vi "GetType.vi"(8 "error in (no error)":errorcluster, 11 "Configure Alarms Msg":refnum<class "Configure Alarms Msg.lvclass">) -> (0 "error out":errorcluster, 2 "Data Sample":variant, 3 "Configure Alarms Msg":refnum<class "Configure Alarms Msg.lvclass">)   [LabVIEW 2015, in "LS218.lvlib" / "Configure Alarms Msg.lvclass"]
uses:
  Configure Alarms Msg.lvclass
  Configure Alarms Msg.lvclass/Configure Alarms Msg.ctl
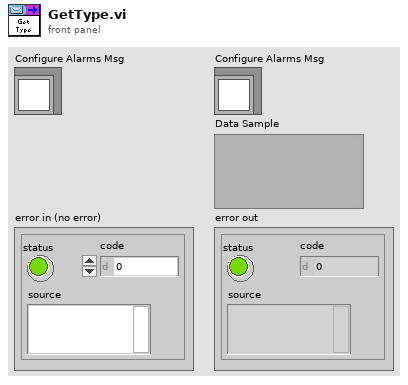
[diagram p1: front panel]
types:
  T1 = cluster{"High Value (0.0000)":dbl[unit], "Low Value (0.0000)":dbl[unit], "Deadband (0.0000)":dbl[unit]}
  T2 = cluster{"Alarm (F: Alarm Disabled)":bool, "Beeper (F: Beeper Disabled)":bool, "Latching (F: Alarm Latch OFF)":bool}
  T3 = cluster{"Input (0)":i32, "Alarm Limits":cluster{"High Value (0.0000)":dbl[unit], "Low Value (0.0000)":dbl[unit], "Deadband (0.0000)":dbl[unit]}, "Boolean Alarm Controls":cluster{"Alarm (F: Alarm Disabled)":bool, "Beeper (F: Beeper Disabled)":bool, "Latching (F: Alarm Latch OFF)":bool}}
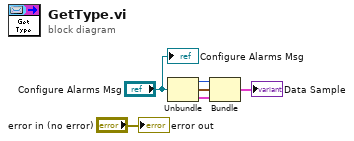
[diagram p0: block diagram]
diagram:
  n1 = Unbundle("Configure Alarms Msg") -> (w3:i32, w2:T1, w1:T2)
  n2 = Bundle("Input (0)"=w3, "Alarm Limits"=w2, "Boolean Alarm Controls"=w1) -> (→"Data Sample":T3)  [unwired: 1 in]
  "error out" <- "error in (no error)"
  "Configure Alarms Msg" <- "Configure Alarms Msg"
